vi "Agilent_33220A_FuncGen_TCP_2.vi"() -> ()   [LabVIEW 2019, in "Models of External Instruments.lvlib"]
uses:
  Models of External Instruments.lvlib
  <vilib>/measure/NI_MABase.lvlib
panel:
  out "error out":errorcluster
  out "Pulse Period":string
  out "Output SYNC Read Buffer":string
  in  "SYNC ON/OFF":bool
  out "Output Waveform Status":string
  out "Output Status":string
  out "Frequency":string
  out "Waveform Type":string
  out "Offset":string
  out "Vpp":string
  out "Waveform Graph":waveform(dbl)(graph)
  out "Result Waveform":string
  out "Waveform Read Buffer":string
  in  "Waveform Generator":enum32{"STATUS", "SIN", "PULSE", "RAMP", "DC"}(tab)
  out "data out":string
  in  "SIN Offset":dbl
  in  "SIN Amplitude":dbl
  in  "SIN Frequency":dbl
  in  "PULSE Amplitude":dbl
  in  "PULSE Offset":dbl
  in  "PULSE Period":dbl
  in  "Pulse Width/Duty Cycle":string(combo)
  in  "PULSE Duty Cycle":dbl
  in  "PULSE Width":dbl
  in  "PULSE Frequency":dbl
  in  "RAMP Frequency":dbl
  in  "RAMP Amplitude":dbl
  in  "RAMP Offset":dbl
  in  "DC Amplitude":dbl
  in  "DC Frequency":dbl
  in  "DC Offset":dbl
  in  "OUTPUT ON/OFF":bool
  out "Output Read Buffer":string
  in  "Stop":bool
  out "bytes written":i32
  # "Output Configuration Commands\n\nOUTP ON\nOUTP OFF \n\nOUTP? --> 1 ON, 0 OFF\n\nOUTP:LOAD? -->yük empedansı\nOUTP:LOAD?  MAX--> maks yük empedansı\nOUTP:LOAD?  MIN--> min yük empedansı\n\nOUTP:POL? --> Normal or Inverted\nOUTP:POL INV -->Inverted waveform\nOUTP:POL?\n\nOUTP:POL NORM-->Normal Waveform\nOUTP:POL?\n\nOUTP:SYNC ON  -->Sync konnectörünü aktif eder\nOUTP:SYNC OFF -->Sync konnectörünü deaktif eder\nOUTP:SYNC? --> Sync konnectörünün durumu 1-ON, 0-OFF\n\nVOLT:UNIT? --> Voltaj biriminin durumu\nVOLT:UNIT VRMS -->birim Vrms\nVOLT:UNIT VPP -->birim Vpp\nVOLT:UNIT DBM -->birim dBm"
  # "Pulse Configuration Commands\n\nPULS:PER 5  --> saniye cinsinden darbe periydunun ayarı\nPULS:PER MIN --> Minimumu 200ns olarak ayarlar\nPULS:PER MAX --> Maxı 2000s olarak ayarlar\nPULS:PER? -*->pulse periyot durumu\n\nFUNC:PULSE:HOLD WIDT --> pulse genişliği şeklinde ayarla\nFUNC:PULSE:HOLD DCYC --> pulse duty cycle şeklinde ayarla\nFUNC:PULSE:HOLD? -->Pulse ayar durumu\n\nFUNC:PULS:WIDT 5-->Pulse genişliği saniye cinsinden ayarla\nFUNC:PULS:WIDT MAX --> Pulse genişliğini max 1999.99 s olarak ayarla\nFUNC:PULS:WIDT MIN --> Pulse genişliğini min 20ns olarak ayarla\nFUNC:PULS:WIDT? --> Pulse genişliğinin durumu\n\nFUNC:PULS:DCYC 50-->Pulse duty cycle'ını oran cinsinden ayarla\nFUNC:PULS:DCYC MAX -->Pulse duty cycle'ını max 100% olarak ayarla\nFUNC:PULS:DCYC MIN --> Pulse duty cycle'ını  min 0% olarak ayarla\nFUNC:PULS:DCYC? -->  Pulse duty cycle'ının durumu\n\nFUNC:PULS:TRAN 50 --> düşen ve yükselen kenar için edge time'ı oran olarak ayarla\n                                             edge time from 5 ns to 100 ns\nFUNC:PULS:TRAN MAX --> edge time 100ns\nFUNC:PULS:TRAN MIN --> edge time 5ns\nFUNC:PULS:TRAN? -->edge time durumu"
  # "APPLy Command\n\nAPPL:SIN 5 KHZ, 3.0 VPP, -2.5 V\nAPPL?\n\nAPPL:SIN 5.0E+3, 3.0 VRMS, -2.5\nAPPL?\n\nAPPL:SQU 5.0E+3, 3.0, -2.5\nAPPL?"
  # "APPLy\n:SINusoid [<frequency> [,<amplitude> [,<offset>] ]]\n:SQUare [<frequency> [,<amplitude> [,<offset>] ]]\n:RAMP [<frequency> [,<amplitude> [,<offset>] ]]\n:PULSe [<frequency> [,<amplitude> [,<offset>] ]]\n:NOISe [<frequency|DEF>1 [,<amplitude> [,<offset>] ]]\n:DC [<frequency|DEF>1 [,<amplitude>|DEF>1 [,<offset>] ]]\n:USER [<frequency> [,<amplitude> [,<offset>] ]]\nAPPLy?"
  # "Low-Level Commands\n\nFUNC SIN --> Select sine wave function\nFREQ 5000 -->Set frequency to 5 kHz\nVOLT 3.0 --> Set amplitude to 3 Vpp\nVOLT:OFFS -2.5 --> Set offset to -2.5 Vdc\nAPPL?"
  # "*IDN? --> cihaz bilgileri: Agilent Technologies,33220A,<serial number>,f.ff-b.bb-aa-p\n                                            f.ff = Firmware revision number\n                                            b.bb = Boot kernel revision number\n                                            aa = ASIC revision number\n                                            p = Printed circuit board revision number\nSYSTem:VERSion? --> sistem verisyonu\n\nSYST:ERR? --> Hataları oku\n\nDISP ON--> ekranı aç\nDISP OFF--> ekranı kapat\nDISP? --> ekran durumu"
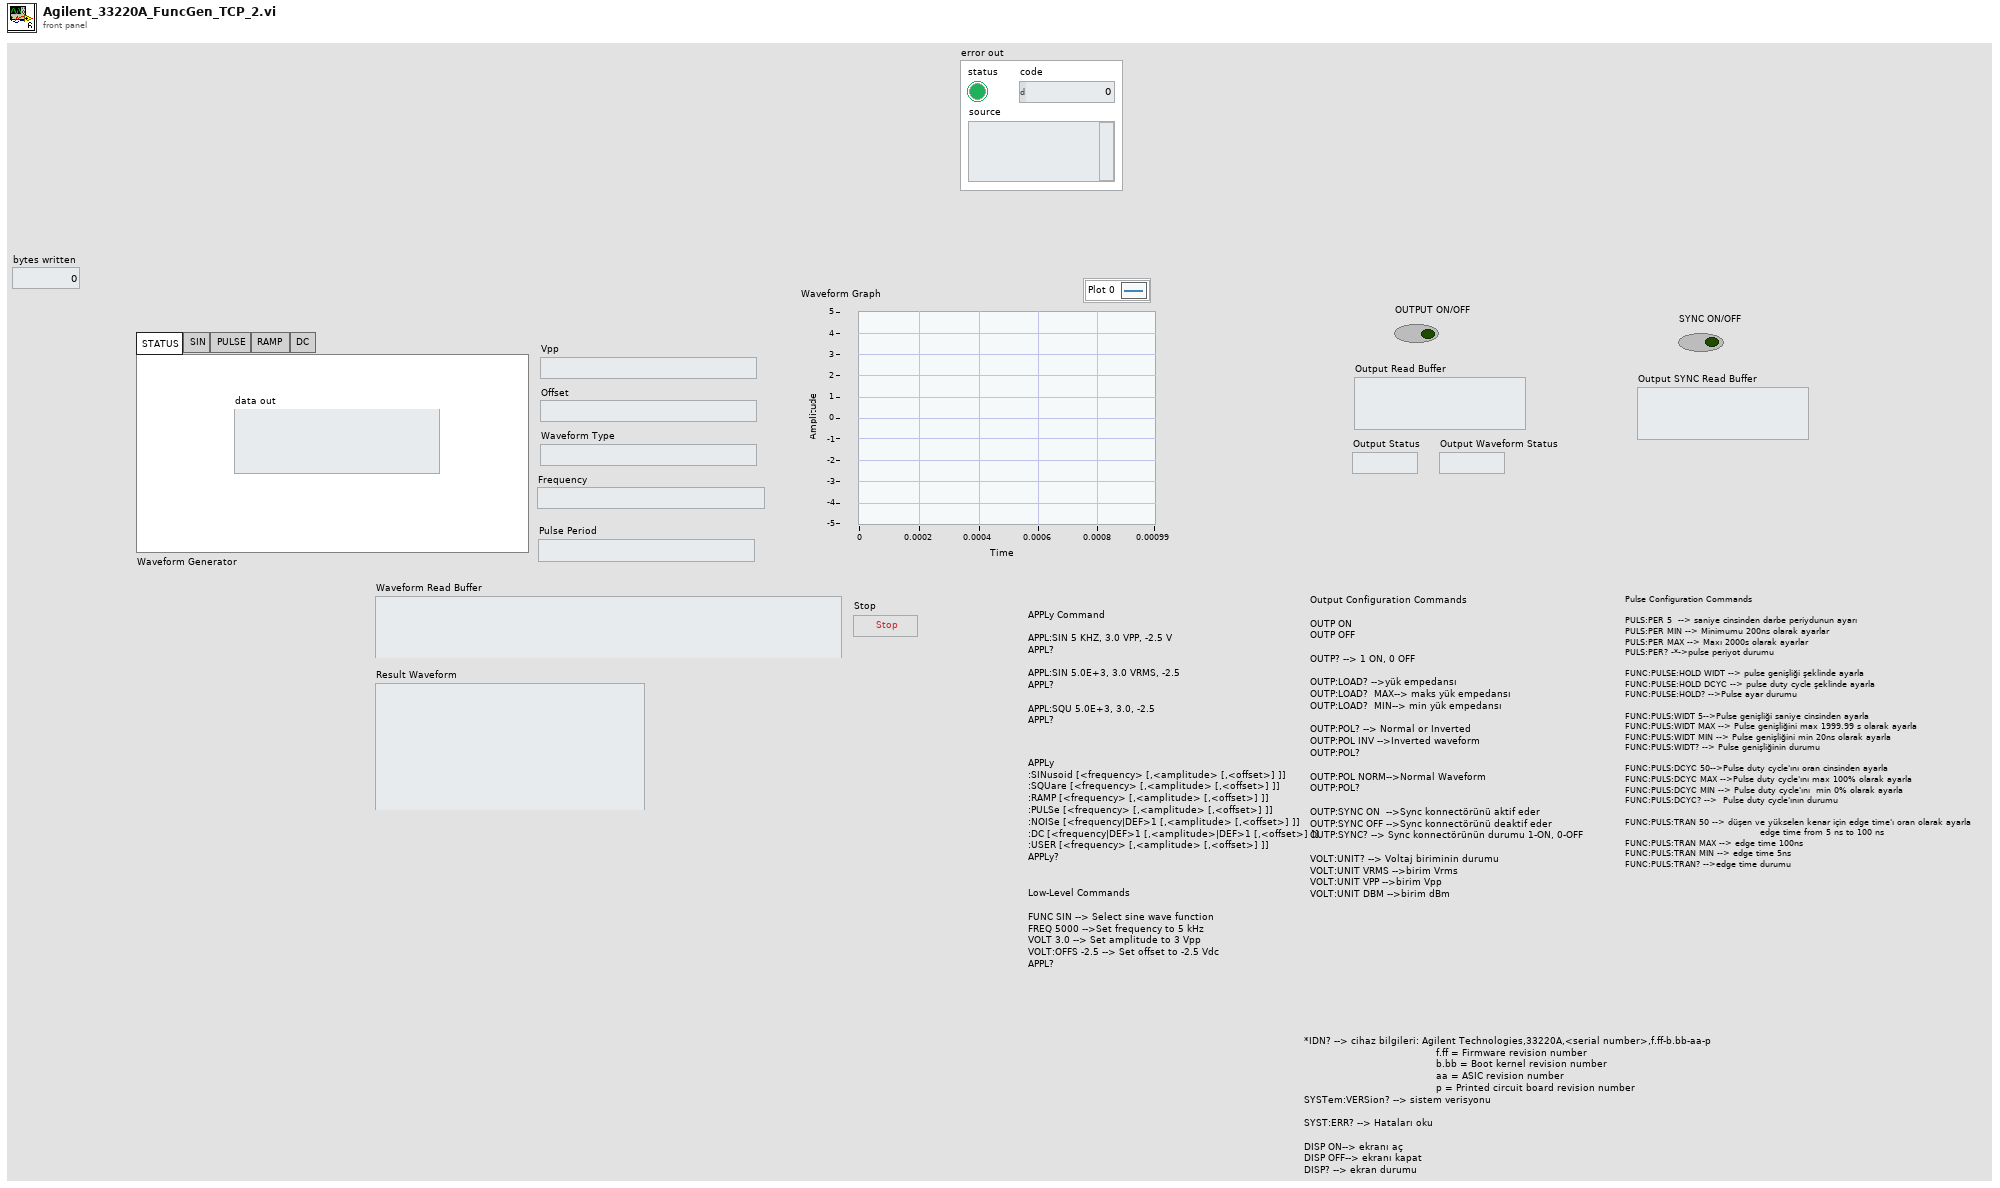
[diagram p1: front panel]
types:
  T1 = enum16{"Sine Wave", "Triangle Wave", "Square Wave", "Sawtooth Wave"}
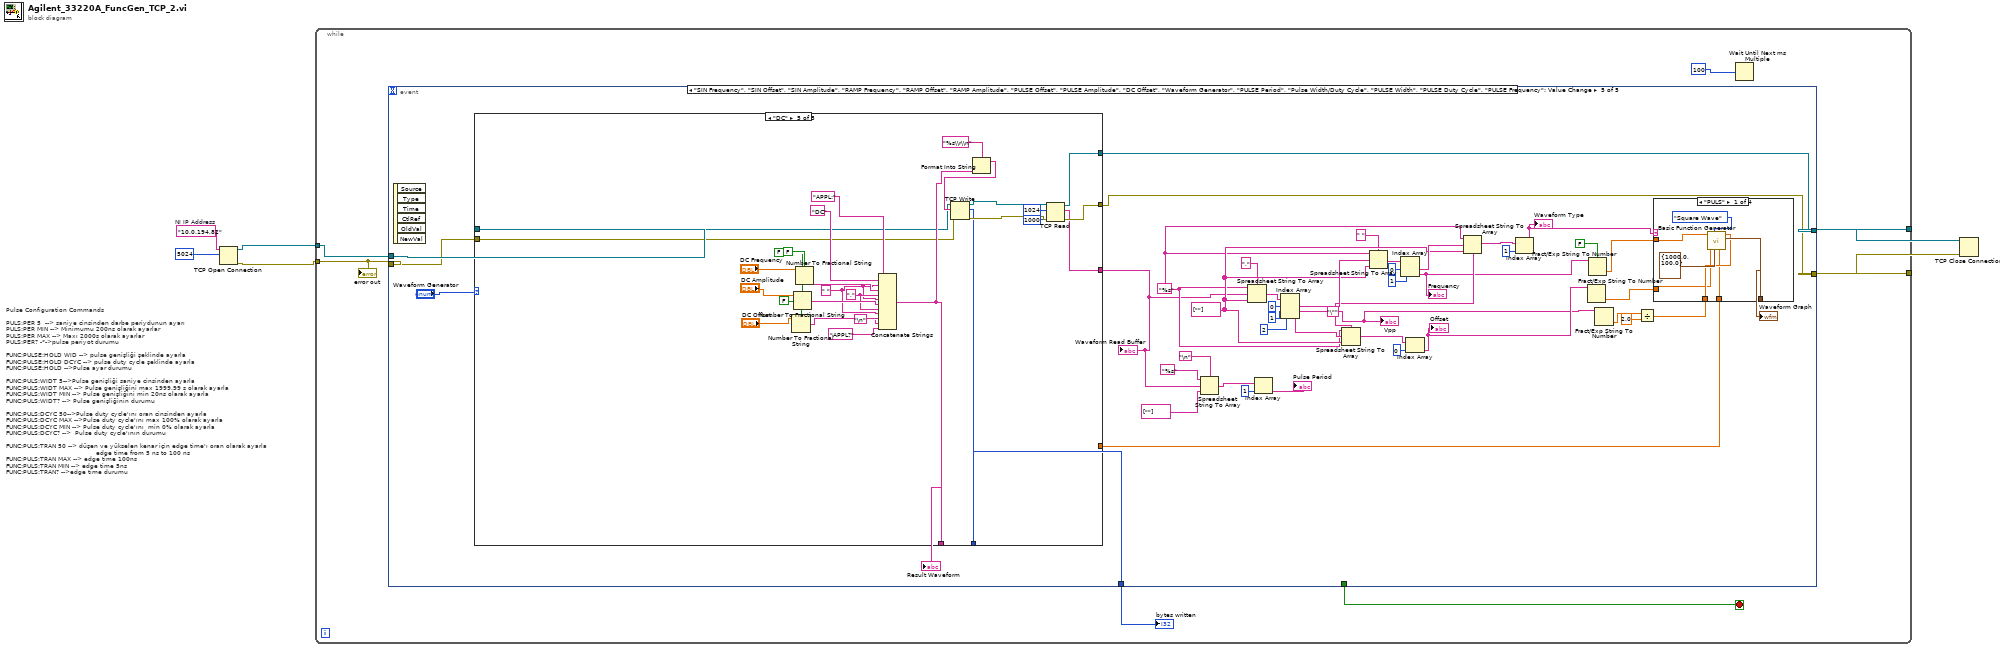
[diagram p0: block diagram]
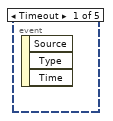
[diagram p2: hidden frame]
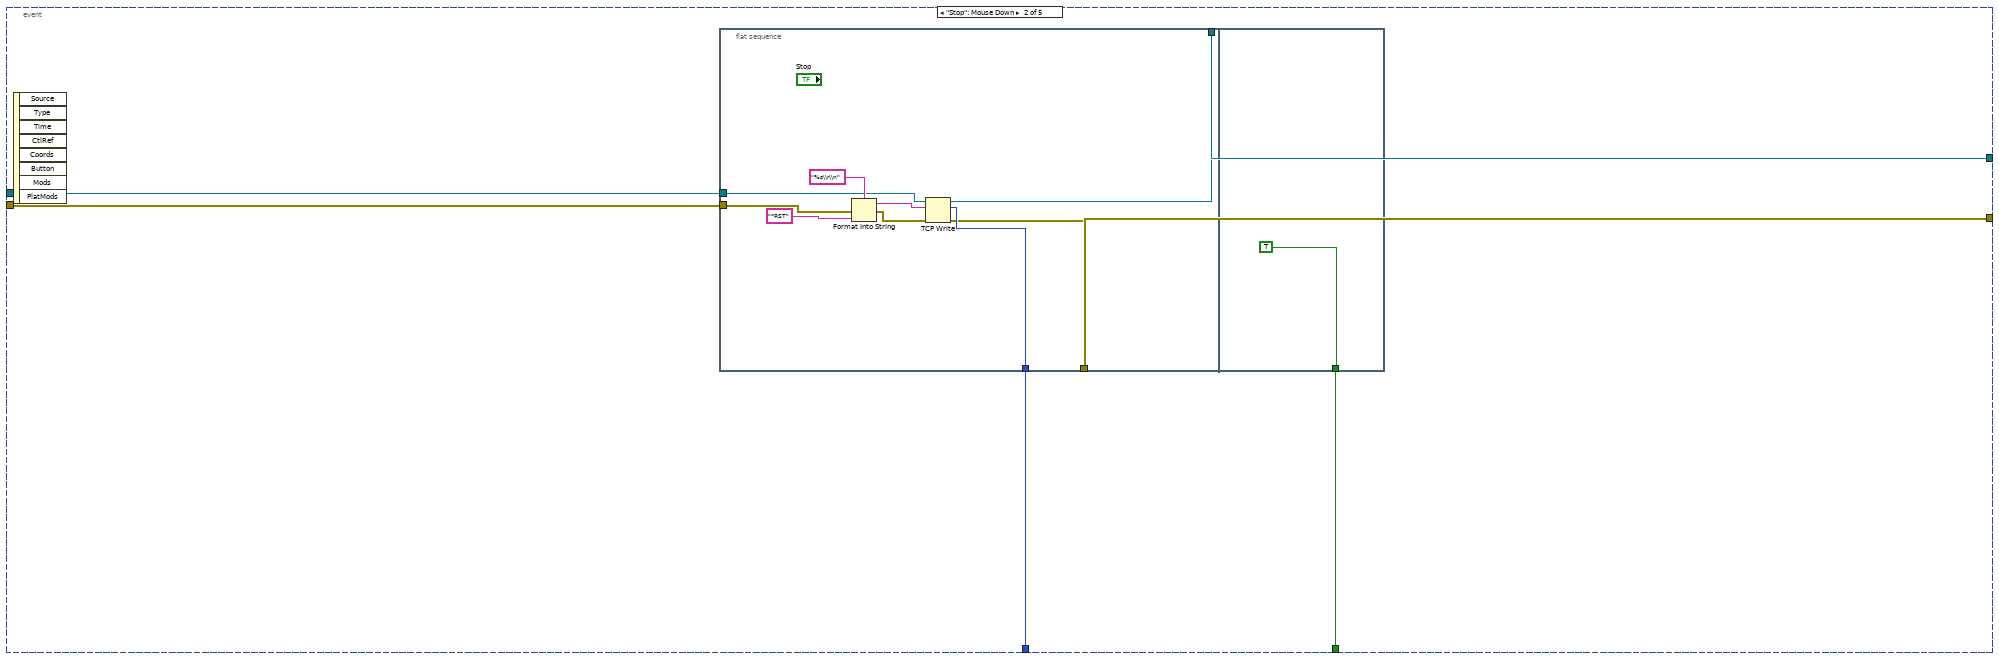
[diagram p3: hidden frame]
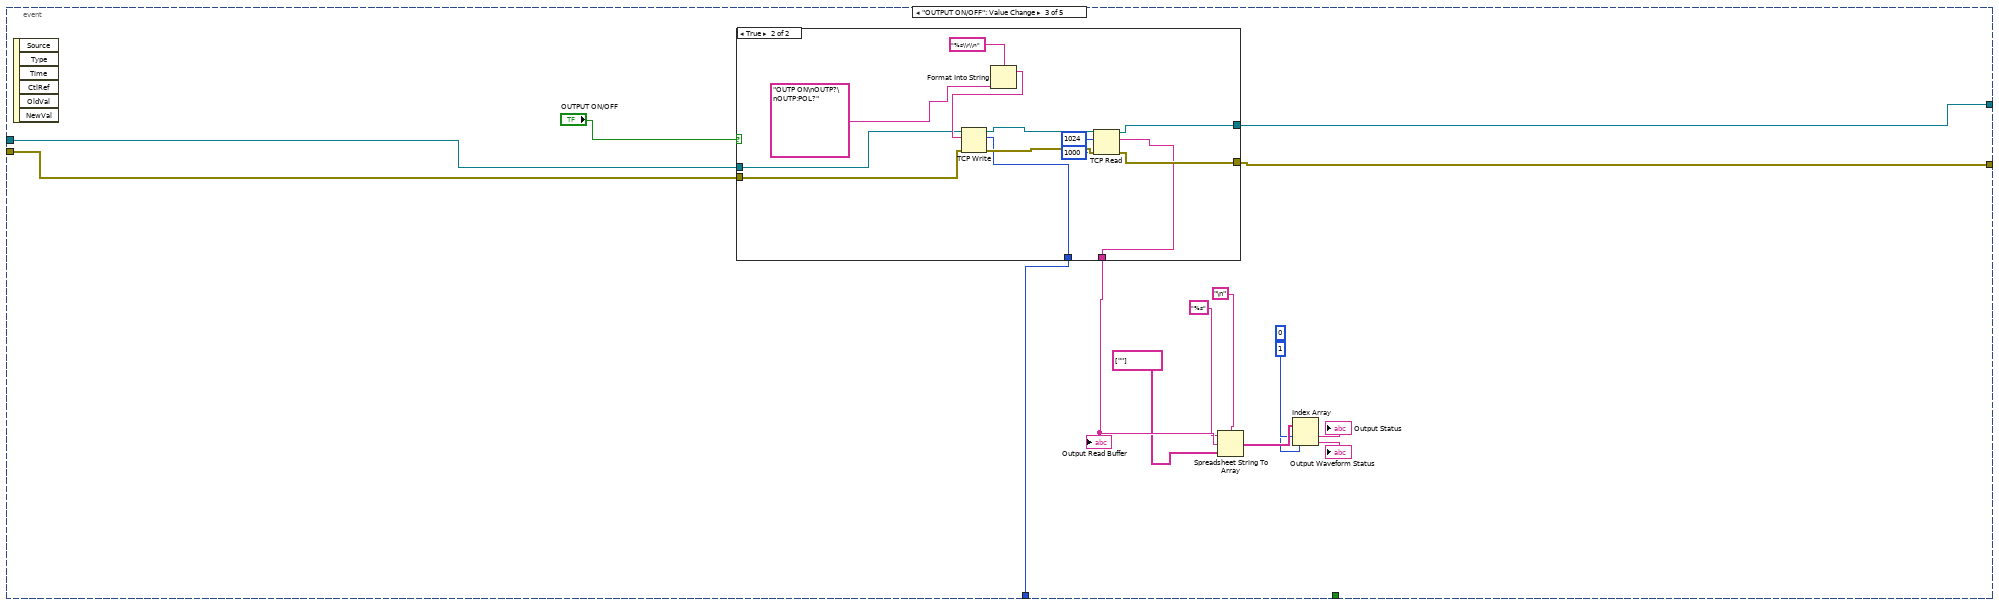
[diagram p4: hidden frame]
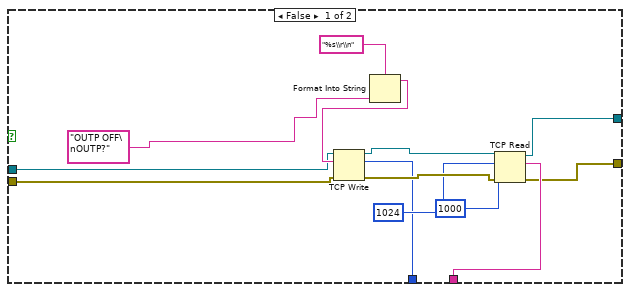
[diagram p5: hidden frame]
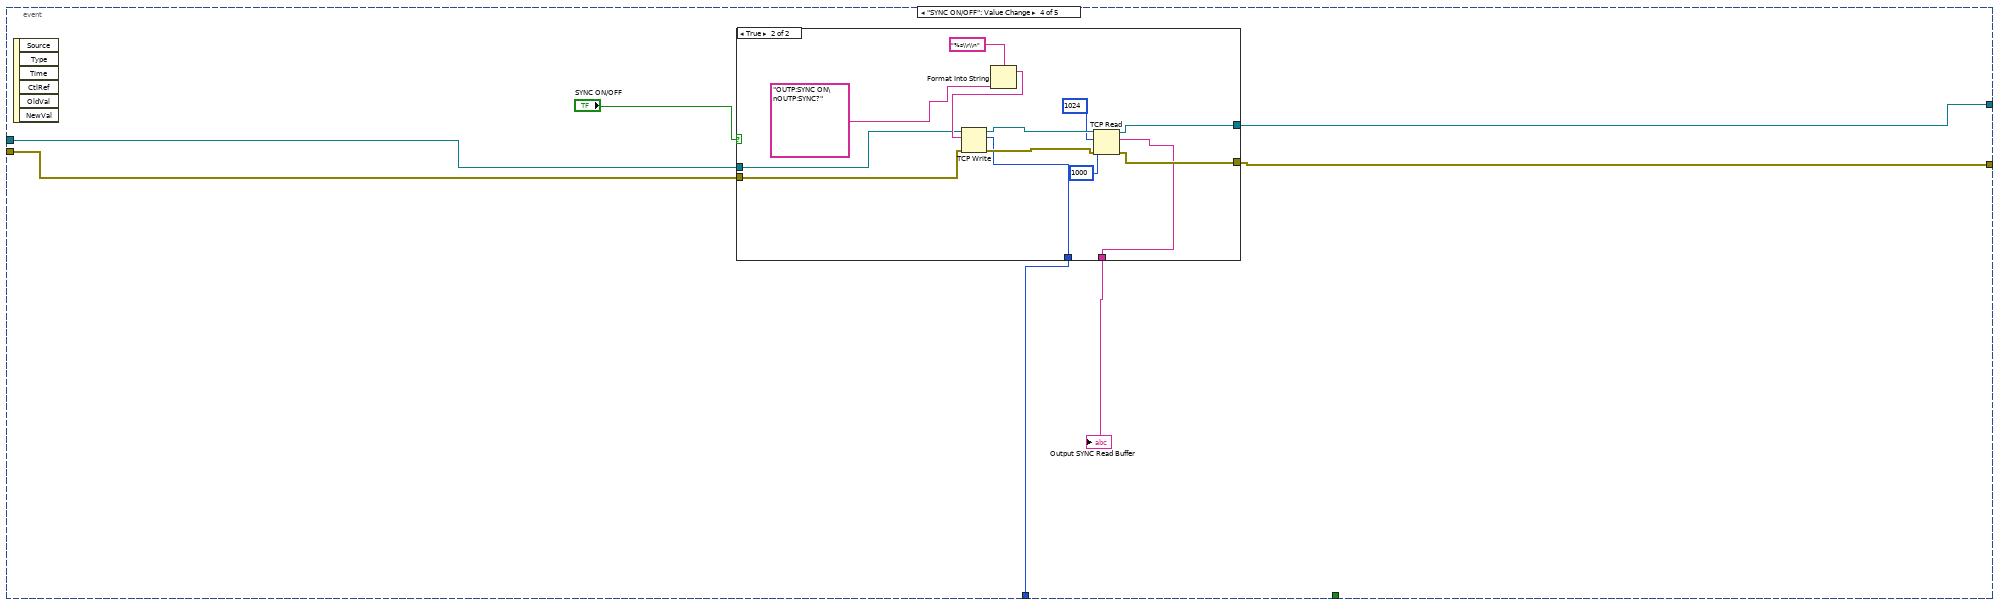
[diagram p6: hidden frame]
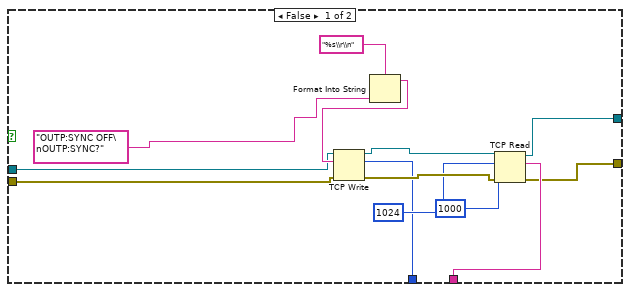
[diagram p7: hidden frame]
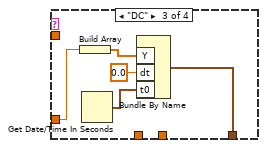
[diagram p9: hidden frame]
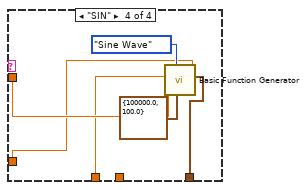
[diagram p10: hidden frame]
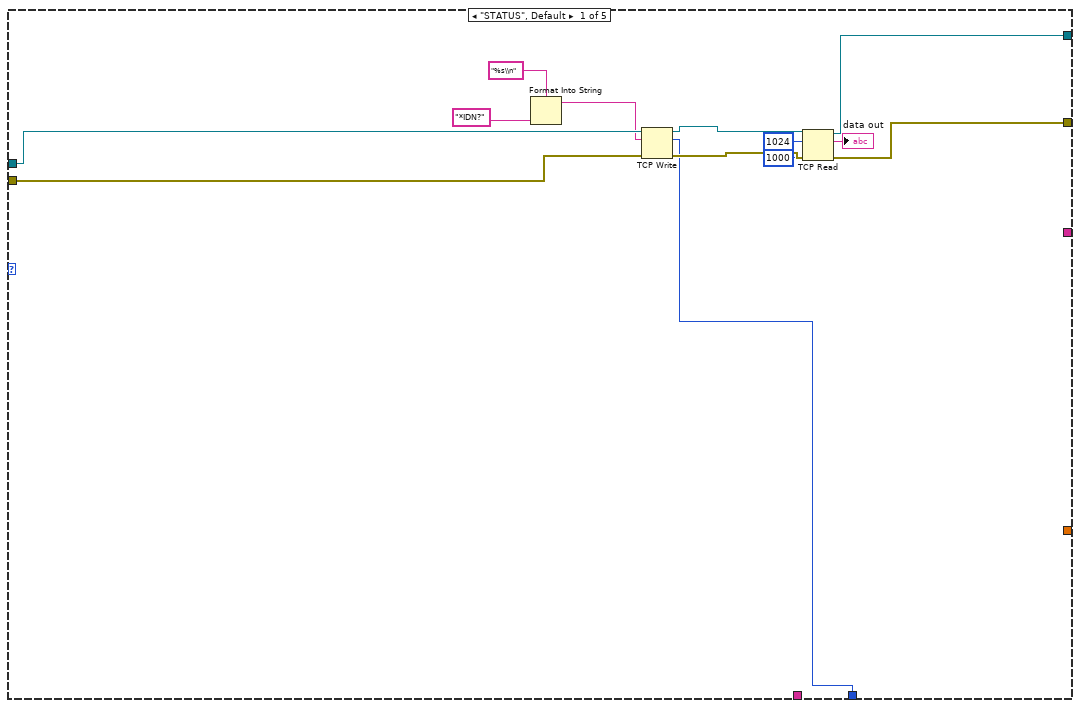
[diagram p11: hidden frame]
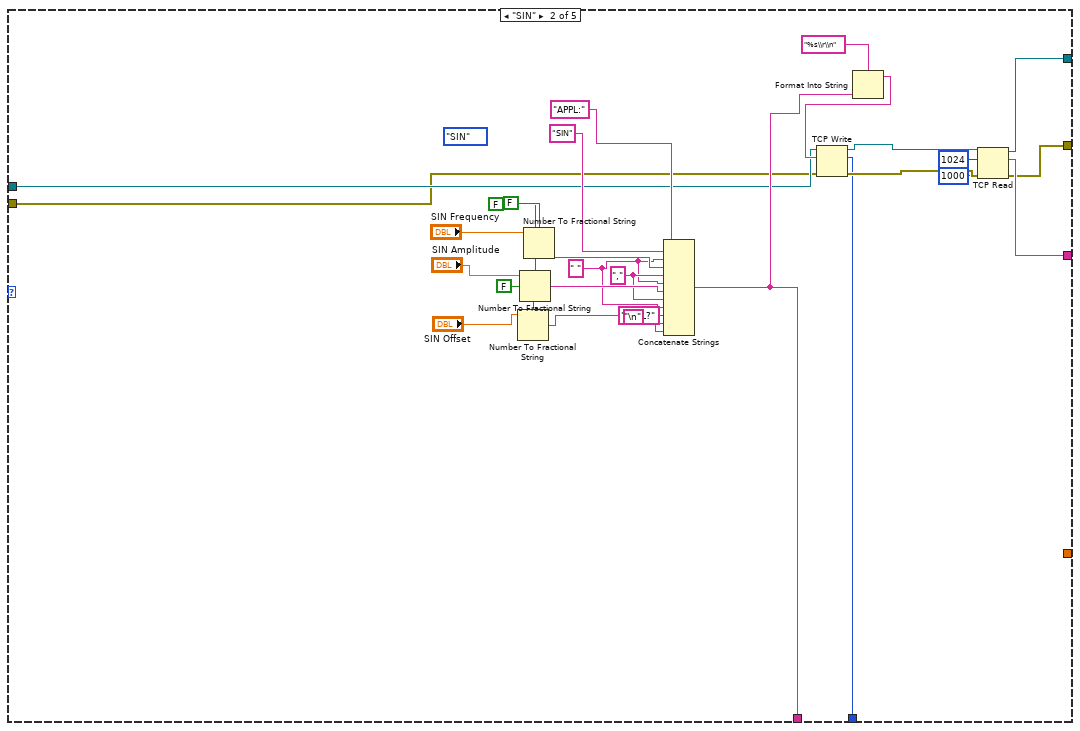
[diagram p12: hidden frame]
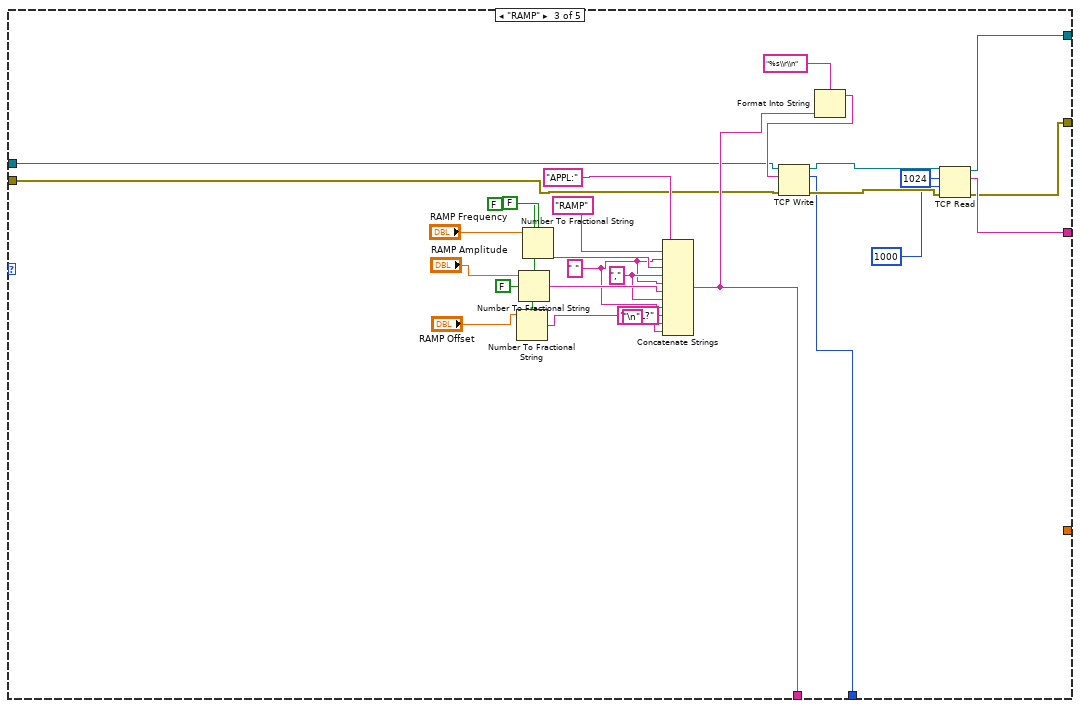
[diagram p13: hidden frame]
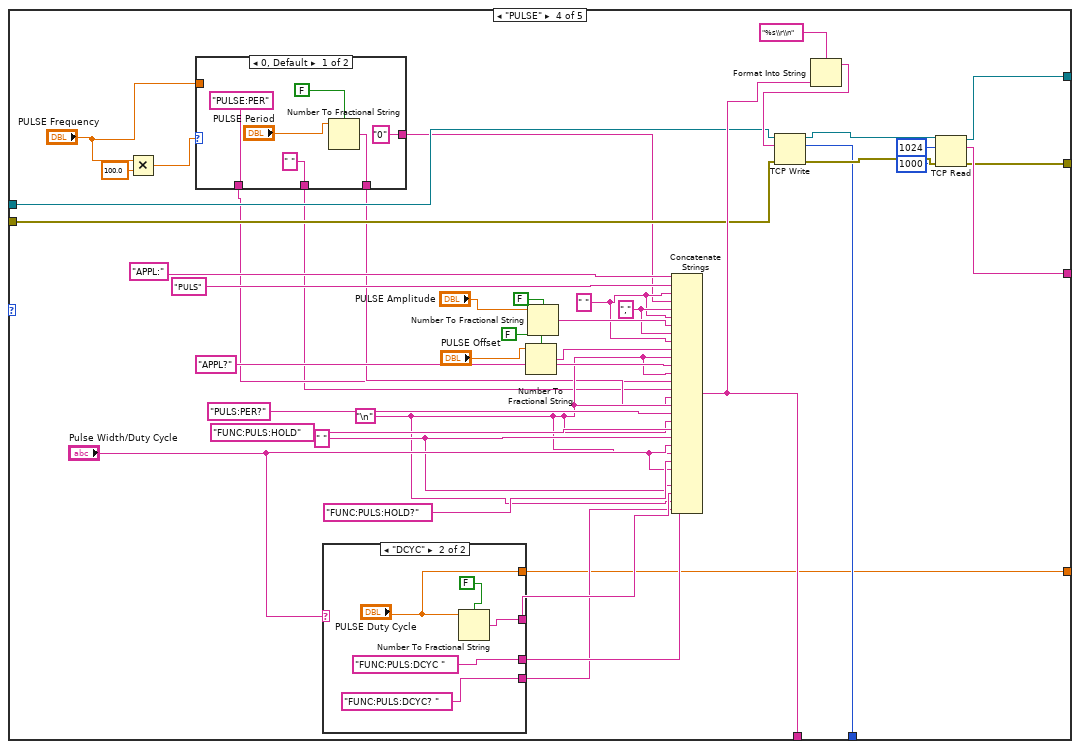
[diagram p14: hidden frame]
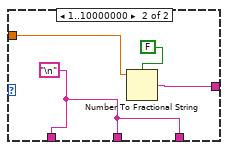
[diagram p15: hidden frame]
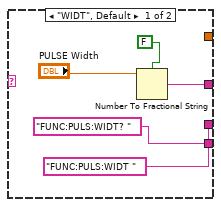
[diagram p16: hidden frame]
diagram:
  w5 = "10.0.194.82"  # NI IP Address
  # "Pulse Configuration Commands\n\nPULS:PER 5  --> saniye cinsinden darbe periydunun ayarı\nPULS:PER MIN --> Minimumu 200ns olarak ayarlar\nPULS:PER MAX --> Maxı 2000s olarak ayarlar\nPULS:PER? -*->pulse periyot durumu\n\nFUNC:PULSE:HOLD WID --> pulse genişliği şeklinde ayarla\nFUNC:PULSE:HOLD DCYC --> pulse duty cycle şeklinde ayarla\nFUNC:PULSE:HOLD -->Pulse ayar durumu\n\nFUNC:PULS:WIDT 5-->Pulse genişliği saniye cinsinden ayarla\nFUNC:PULS:WIDT MAX --> Pulse genişliğini max 1999.99 s olarak ayarla\nFUNC:PULS:WIDT MIN --> Pulse genişliğini min 20ns olarak ayarla\nFUNC:PULS:WIDT? --> Pulse genişliğinin durumu\n\nFUNC:PULS:DCYC 50-->Pulse duty cycle'ını oran cinsinden ayarla\nFUNC:PULS:DCYC MAX -->Pulse duty cycle'ını max 100% olarak ayarla\nFUNC:PULS:DCYC MIN --> Pulse duty cycle'ını  min 0% olarak ayarla\nFUNC:PULS:DCYC? -->  Pulse duty cycle'ının durumu\n\nFUNC:PULS:TRAN 50 --> düşen ve yükselen kenar için edge time'ı oran olarak ayarla\n                                             edge time from 5 ns to 100 ns\nFUNC:PULS:TRAN MAX --> edge time 100ns\nFUNC:PULS:TRAN MIN --> edge time 5ns\nFUNC:PULS:TRAN? -->edge time durumu"
  n1 = TCP Open Connection(address=w5, remote port or service name=u16 5024 ("port or service name")) -> (connection ID=w4:refnum<k5>, error out=w3:errorcluster)  [unwired: 3 in]
  n2 = while {
    tunnel: w4 -> [w12]
    tunnel: w3 -> [w11]
    tunnel: [w10] -> w2
    tunnel: [w9] -> w1
    stop <- w7 stop-if-true
    n3 = event shown="[4] \"SIN Frequency\", \"SIN Offset\", \"SIN Amplitude\", \"RAMP Frequency\", \"RAMP Offset\", \"RAMP Amplitude\", \"PULSE Offset\", \"PULSE Amplitude\", \"DC Offset\", \"Waveform Generator\", \"PULSE Period\", \"Pulse Width/Duty Cycle\", \"PULSE Width\", \"PULSE Duty Cycle\", \"PULSE Frequency\": Value Change" {
      selector: _ -> [_ _ _ _ _]
      dyn-events: _ -> [_ _ _ _ _]
      timeout: _ -> [_ _ _ _ _]
      tunnel: w12 -> [_ w19 w43 w77 w117]
      tunnel: w11 -> [_ w18 w42 w76 w116]
      tunnel: [_ w17 w40 w74 w115] -> w10
      tunnel: [_ w16 w39 w73 w114] -> w9
      tunnel: [_ w15 w41 w75 w106] -> w8
      tunnel: [_ w14 _ _ _] -> w7
      event Timeout {
        n4 = event-data() -> ()  [unwired: 1 in, 3 out]
      }
      event "Stop": Mouse Down {
        n5 = event-data() -> ()  [unwired: 1 in, 8 out]
        n6 = flat-sequence {
          tunnel: [w25] -> w15
          tunnel: w19 -> [w23]
          tunnel: w18 -> [w22]
          tunnel: [w21] -> w17
          tunnel: [w20] -> w16
          tunnel: [TRUE] -> w14
          frame #0 {
            n7 = Format Into String(format string="%s\\r\\n", error in=w22, "*RST" ("input 1")) -> (resulting string=w27:string, error out=w24:errorcluster)  [unwired: 1 in]
            n8 = TCP Write(connection ID=w23, data in=w27, error in (no error)=w24) -> (connection ID out=w21:refnum<k5>, bytes written=w25:i32, error out=w20:errorcluster)  [unwired: 1 in]
          }
          frame #1 {
          }
        }
      }
      event "OUTPUT ON/OFF": Value Change {
        n9 = event-data() -> ()  [unwired: 1 in, 6 out]
        n10 = case shown="True" "OUTPUT ON/OFF" {
          tunnel: [w51 w62] -> w38
          tunnel: [w50 w64] -> w40
          tunnel: [w49 w63] -> w39
          tunnel: [w48 w61] -> w41
          tunnel: w43 -> [w46 w59]
          tunnel: w42 -> [w45 w58]
          frame False {
            n11 = Format Into String(format string="%s\\r\\n", "OUTP OFF\nOUTP?" ("write buffer")) -> (resulting string=w57:string)  [unwired: 2 in, 1 out]
            n12 = TCP Write(connection ID=w46, data in=w57, error in (no error)=w45) -> (connection ID out=w55:refnum<k5>, bytes written=w48:i32, error out=w56:errorcluster)  [unwired: 1 in]
            n13 = TCP Read(connection ID=w55, bytes to read=1024, error in (no error)=w56, 9:1000 ("timeout ms (25000)")) -> (connection ID out=w50:refnum<k5>, data out=w51:string, error out=w49:errorcluster)  [unwired: 1 in]
          }
          frame True {
            n14 = Format Into String(format string="%s\\r\\n", "OUTP ON\nOUTP?\nOUTP:POL?" ("write buffer")) -> (resulting string=w70:string)  [unwired: 2 in, 1 out]
            n15 = TCP Write(connection ID=w59, data in=w70, error in (no error)=w58) -> (connection ID out=w68:refnum<k5>, bytes written=w61:i32, error out=w69:errorcluster)  [unwired: 1 in]
            n16 = TCP Read(connection ID=w68, bytes to read=1024, error in (no error)=w69, 9:1000 ("timeout ms (25000)")) -> (connection ID out=w64:refnum<k5>, data out=w62:string, error out=w63:errorcluster)  [unwired: 1 in]
          }
        }
        "Output Read Buffer" <- w38
        n17 = Spreadsheet String To Array(delimiter (Tab)="\n", format string="%s", spreadsheet string=w38, array type (2D Dbl)=string[] [""]) -> (array=w34:string[])
        n18 = Index Array(array=w34, index #1=0 ("index"), index #2=1 ("index")) -> (element #1=→"Output Status":string, element #2=→"Output Waveform Status":string)
      }
      event "SYNC ON/OFF": Value Change {
        n19 = event-data() -> ()  [unwired: 1 in, 6 out]
        n20 = case shown="True" "SYNC ON/OFF" {
          tunnel: [w84 w95] -> w72
          tunnel: [w83 w97] -> w74
          tunnel: [w82 w96] -> w73
          tunnel: [w81 w94] -> w75
          tunnel: w77 -> [w79 w92]
          tunnel: w76 -> [w78 w91]
          frame False {
            n21 = Format Into String(format string="%s\\r\\n", "OUTP:SYNC OFF\nOUTP:SYNC?" ("write buffer")) -> (resulting string=w90:string)  [unwired: 2 in, 1 out]
            n22 = TCP Write(connection ID=w79, data in=w90, error in (no error)=w78) -> (connection ID out=w88:refnum<k5>, bytes written=w81:i32, error out=w89:errorcluster)  [unwired: 1 in]
            n23 = TCP Read(connection ID=w88, bytes to read=1024, error in (no error)=w89, 9:1000 ("timeout ms (25000)")) -> (connection ID out=w83:refnum<k5>, data out=w84:string, error out=w82:errorcluster)  [unwired: 1 in]
          }
          frame True {
            n24 = Format Into String(format string="%s\\r\\n", "OUTP:SYNC ON\nOUTP:SYNC?" ("write buffer")) -> (resulting string=w103:string)  [unwired: 2 in, 1 out]
            n25 = TCP Write(connection ID=w92, data in=w103, error in (no error)=w91) -> (connection ID out=w101:refnum<k5>, bytes written=w94:i32, error out=w102:errorcluster)  [unwired: 1 in]
            n26 = TCP Read(connection ID=w101, bytes to read=1024, error in (no error)=w102, 9:1000 ("timeout ms (25000)")) -> (connection ID out=w97:refnum<k5>, data out=w95:string, error out=w96:errorcluster)  [unwired: 1 in]
          }
        }
        "Output SYNC Read Buffer" <- w72
      }
      event "SIN Frequency", "SIN Offset", "SIN Amplitude", "RAMP Frequency", "RAMP Offset", "RAMP Amplitude", "PULSE Offset", "PULSE Amplitude", "DC Offset", "Waveform Generator", "PULSE Period", "Pulse Width/Duty Cycle", "PULSE Width", "PULSE Duty Cycle", "PULSE Frequency": Value Change {
        w140 = "\"" ("delimiter (Tab)")
        w139 = string[] [""]
        w138 = "%s" ("format string")
        n27 = event-data() -> ()  [unwired: 1 in, 6 out]
        n28 = case shown="\"DC\"" "Waveform Generator" {
          tunnel: [_ w185 w212 w258 w299] -> w113
          tunnel: [_ w186 w214 w259 w303] -> w124
          tunnel: [w175 w183 w211 w257 w301] -> w115
          tunnel: [w174 w182 w210 w256 w300] -> w114
          tunnel: [w167 w184 w213 w255 w302] -> w106
          tunnel: w117 -> [w173 w181 w209 w254 w298]
          tunnel: w116 -> [w168 w180 w208 w253 w297]
          tunnel: [_ _ _ w236 _] -> w105
          frame "STATUS", Default {
            n29 = Format Into String(format string="%s\\n", "*IDN?" ("data in")) -> (resulting string=w169:string)  [unwired: 2 in, 1 out]
            n30 = TCP Write(connection ID=w173, data in=w169, error in (no error)=w168) -> (connection ID out=w178:refnum<k5>, bytes written=w167:i32, error out=w179:errorcluster)  [unwired: 1 in]
            n31 = TCP Read(connection ID=w178, bytes to read=1024, error in (no error)=w179, 9:1000 ("timeout ms (25000)")) -> (connection ID out=w175:refnum<k5>, data out=→"data out":string, error out=w174:errorcluster)  [unwired: 1 in]
          }
          frame "SIN" {
            w196 = " " ("string")
            (unwired) enum32{"SIN", "PULSE", "RAMP", "DC"}."SIN" ("Tab Control")
            w199 = "," ("string")
            n32 = Number To Fractional String(use system decimal point (T)=FALSE, number="SIN Offset") -> (F-format string=w205:string)  [unwired: 2 in]
            n33 = Number To Fractional String(use system decimal point (T)=FALSE, number="SIN Amplitude") -> (F-format string=w204:string)  [unwired: 2 in]
            n34 = Number To Fractional String(use system decimal point (T)=FALSE, number="SIN Frequency") -> (F-format string=w202:string)  [unwired: 2 in]
            n35 = Concatenate Strings("APPL:", "SIN", w196, w202, w199, w196, w204, w199, w196, w205, "\n", "APPL?" ("string")) -> (w186:string)
            n36 = Format Into String(format string="%s\\r\\n", w186) -> (resulting string=w192:string)  [unwired: 2 in, 1 out]
            n37 = TCP Write(connection ID=w181, data in=w192, error in (no error)=w180) -> (connection ID out=w190:refnum<k5>, bytes written=w184:i32, error out=w191:errorcluster)  [unwired: 1 in]
            n38 = TCP Read(connection ID=w190, bytes to read=1024, error in (no error)=w191, 9:1000 ("timeout ms (25000)")) -> (connection ID out=w183:refnum<k5>, data out=w185:string, error out=w182:errorcluster)  [unwired: 1 in]
          }
          frame "RAMP" {
            w225 = " " ("string")
            w228 = "," ("string")
            n39 = Number To Fractional String(use system decimal point (T)=FALSE, number="RAMP Offset") -> (F-format string=w233:string)  [unwired: 2 in]
            n40 = Number To Fractional String(use system decimal point (T)=FALSE, number="RAMP Amplitude") -> (F-format string=w232:string)  [unwired: 2 in]
            n41 = Number To Fractional String(use system decimal point (T)=FALSE, number="RAMP Frequency") -> (F-format string=w230:string)  [unwired: 2 in]
            n42 = Concatenate Strings("APPL:", "RAMP", w225, w230, w228, w225, w232, w228, w225, w233, "\n", "APPL?" ("string")) -> (w214:string)
            n43 = Format Into String(format string="%s\\r\\n", w214) -> (resulting string=w220:string)  [unwired: 2 in, 1 out]
            n44 = TCP Write(connection ID=w209, data in=w220, error in (no error)=w208) -> (connection ID out=w218:refnum<k5>, bytes written=w213:i32, error out=w219:errorcluster)  [unwired: 1 in]
            n45 = TCP Read(connection ID=w218, bytes to read=1024, error in (no error)=w219, 9:1000 ("timeout ms (25000)")) -> (connection ID out=w211:refnum<k5>, data out=w212:string, error out=w210:errorcluster)  [unwired: 1 in]
          }
          frame "PULSE" {
            w247 = " " ("string")
            w245 = "\n"
            w269 = " " ("string")
            w271 = "," ("string")
            n46 = Multiply(x="PULSE Frequency", y=100.0) -> (x*y=w239:dbl)
            n47 = case shown="0, Default" w239 {
              tunnel: [w282 w285] -> w243
              tunnel: ["PULSE:PER" ("string") w285] -> w242
              tunnel: [" " ("string") w285] -> w241
              tunnel: "PULSE Frequency" -> [_ w284]
              tunnel: ["0" w283] -> w237
              frame 0, Default {
                n48 = Number To Fractional String(use system decimal point (T)=FALSE, number="PULSE Period") -> (F-format string=w282:string)  [unwired: 2 in]
              }
              frame 1..10000000 {
                w285 = "\n"
                n49 = Number To Fractional String(use system decimal point (T)=FALSE, number=w284) -> (F-format string=w283:string)  [unwired: 2 in]
              }
            }
            n50 = case shown="\"DCYC\"" "Pulse Width/Duty Cycle" {
              tunnel: ["FUNC:PULS:WIDT " ("string") "FUNC:PULS:DCYC " ("string")] -> w248
              tunnel: [w288 w295] -> w246
              tunnel: ["FUNC:PULS:WIDT? " ("string") "FUNC:PULS:DCYC? " ("string")] -> w244
              tunnel: [_ "PULSE Duty Cycle"] -> w236
              frame "WIDT", Default {
                n51 = Number To Fractional String(use system decimal point (T)=FALSE, number="PULSE Width") -> (F-format string=w288:string)  [unwired: 2 in]
              }
              frame "DCYC" {
                n52 = Number To Fractional String(use system decimal point (T)=FALSE, number="PULSE Duty Cycle") -> (F-format string=w295:string)  [unwired: 2 in]
              }
            }
            n53 = Number To Fractional String(use system decimal point (T)=FALSE, number="PULSE Offset") -> (F-format string=w274:string)  [unwired: 2 in]
            n54 = Number To Fractional String(use system decimal point (T)=FALSE, number="PULSE Amplitude") -> (F-format string=w273:string)  [unwired: 2 in]
            n55 = Concatenate Strings("APPL:", "PULS", w269, w237, w271, w269, w273, w271, w269, w274, w245, "APPL?" ("string"), w245, w242, w241, w243, w245, "PULS:PER?" ("string"), w245, "FUNC:PULS:HOLD" ("string"), w247, "Pulse Width/Duty Cycle", w245, "FUNC:PULS:HOLD?" ("string"), w245, w248, w247, w246, w245, w244) -> (w259:string)
            n56 = Format Into String(format string="%s\\r\\n", w259) -> (resulting string=w264:string)  [unwired: 2 in, 1 out]
            n57 = TCP Write(connection ID=w254, data in=w264, error in (no error)=w253) -> (connection ID out=w262:refnum<k5>, bytes written=w255:i32, error out=w263:errorcluster)  [unwired: 1 in]
            n58 = TCP Read(connection ID=w262, bytes to read=1024, error in (no error)=w263, 9:1000 ("timeout ms (25000)")) -> (connection ID out=w257:refnum<k5>, data out=w258:string, error out=w256:errorcluster)  [unwired: 1 in]
          }
          frame "DC" {
            w314 = " " ("string")
            w317 = "," ("string")
            n59 = Number To Fractional String(use system decimal point (T)=FALSE, number="DC Offset") -> (F-format string=w322:string)  [unwired: 2 in]
            n60 = Number To Fractional String(use system decimal point (T)=FALSE, number="DC Amplitude") -> (F-format string=w321:string)  [unwired: 2 in]
            n61 = Number To Fractional String(use system decimal point (T)=FALSE, number="DC Frequency") -> (F-format string=w319:string)  [unwired: 2 in]
            n62 = Concatenate Strings("APPL:", "DC", w314, w319, w317, w314, w321, w317, w314, w322, "\n", "APPL?" ("string")) -> (w303:string)
            n63 = Format Into String(format string="%s\\r\\n", w303) -> (resulting string=w309:string)  [unwired: 2 in, 1 out]
            n64 = TCP Write(connection ID=w298, data in=w309, error in (no error)=w297) -> (connection ID out=w307:refnum<k5>, bytes written=w302:i32, error out=w308:errorcluster)  [unwired: 1 in]
            n65 = TCP Read(connection ID=w307, bytes to read=1024, error in (no error)=w308, 9:1000 ("timeout ms (25000)")) -> (connection ID out=w301:refnum<k5>, data out=w299:string, error out=w300:errorcluster)  [unwired: 1 in]
          }
        }
        "Waveform Read Buffer" <- w113
        "Result Waveform" <- w124
        n66 = Spreadsheet String To Array(delimiter (Tab)="\n", format string="%s", spreadsheet string=w113, array type (2D Dbl)=string[] [""]) -> (array=w109:string[])
        n67 = Spreadsheet String To Array(delimiter (Tab)=",", format string=w138, spreadsheet string=w113, array type (2D Dbl)=w139) -> (array=w141:string[])
        n68 = Index Array(array=w109, index=1) -> (element=→"Pulse Period":string)
        n69 = Index Array(array=w141, index #1=0 ("index"), index #2=1 ("index"), index #3=2 ("index")) -> (element #1=w142:string, element #2=w127:string, element #3=w144:string)
        "Vpp" <- w127
        n70 = Spreadsheet String To Array(delimiter (Tab)=w140, format string=w138, spreadsheet string=w144, array type (2D Dbl)=w139) -> (array=w145:string[])
        n71 = Spreadsheet String To Array(delimiter (Tab)=" ", format string=w138, spreadsheet string=w142, array type (2D Dbl)=w139) -> (array=w143:string[])
        n72 = Index Array(array=w143, index #1=0 ("index"), index #2=1 ("index")) -> (element #1=w146:string, element #2=w126:string)
        "Frequency" <- w126
        n73 = Index Array(array=w145, index=0) -> (element=w128:string)
        "Offset" <- w128
        n74 = Spreadsheet String To Array(delimiter (Tab)=w140, format string=w138, spreadsheet string=w146, array type (2D Dbl)=w139) -> (array=w147:string[])
        n75 = Index Array(array=w147, index=1) -> (element=w125:string)
        "Waveform Type" <- w125
        n76 = Fract/Exp String To Number(string=w128) -> (number=w118:dbl)  [unwired: 3 in, 1 out]
        n77 = Fract/Exp String To Number(use system decimal point (T)=FALSE, string=w126) -> (number=w120:dbl)  [unwired: 2 in, 1 out]
        n78 = Fract/Exp String To Number(string=w127) -> (number=w121:dbl)  [unwired: 3 in, 1 out]
        n79 = Divide(x=w121, y=2.0) -> (x/y=w119:dbl)
        n80 = case shown="\"PULS\"" w125 {
          tunnel: [w154 _ w159 w165] -> w122
          tunnel: w120 -> [w152 _ _ w164]
          tunnel: w119 -> [w151 _ _ w162]
          tunnel: w118 -> [w150 _ w156 w163]
          tunnel: w105 -> [w149 _ _ _]
          frame "PULS" {
            n81 = call <vilib>:"Basic Function Generator.vi"("offset"=w151, "square wave duty cycle (%)"=w149, "sampling info"=cluster{"Fs":dbl, "#s":dbl} {"Fs"=1000.0, "#s"=100.0}, "signal type"=T1."Square Wave", "amplitude"=w150, "frequency"=w152) -> ("signal out"=w154:waveform(dbl))  [unwired: 3 in, 2 out]
          }
          frame Default {
          }
          frame "DC" {
            n82 = Build Array(w156) -> (w160:dbl[])
            n83 = Get Date/Time In Seconds() -> (seconds since 1Jan1904=w157:timestamp)
            n84 = Bundle By Name("Y"=w160, "dt"=0.0, "t0"=w157) -> (w159:waveform(dbl))  [unwired: 1 in]
          }
          frame "SIN" {
            n85 = call <vilib>:"Basic Function Generator.vi"("offset"=w163, "sampling info"=cluster{"Fs":dbl, "#s":dbl} {"Fs"=100000.0, "#s"=100.0}, "signal type"=T1."Sine Wave", "amplitude"=w162, "frequency"=w164) -> ("signal out"=w165:waveform(dbl))  [unwired: 4 in, 2 out]
          }
        }
        "Waveform Graph" <- w122
      }
    }
    "bytes written" <- w8
    n86 = Wait Until Next ms Multiple(millisecond multiple=u32 100) -> ()  [unwired: 1 out]
    "error out" <- w11
  }
  n87 = TCP Close Connection(connection ID=w2, error in (no error)=w1) -> ()  [unwired: 1 in, 2 out]
